vi "Update INI key to users last set value for Boolean.vi"(8 "error in (no error)":errorcluster, 9 "TF for INI (in)":bool, 10 "INI Key":string, 11 "INI Section":string) -> (0 "error out":errorcluster, 1 "TF for INI (out)":bool)   [LabVIEW 2010]
uses:
  <vilib>/Utility/sysdir.llb/System Directory Type.ctl
  <vilib>/Utility/config.llb/Write Key (Boolean).vi
  <vilib>/Utility/config.llb/NI_LVConfig.lvlib
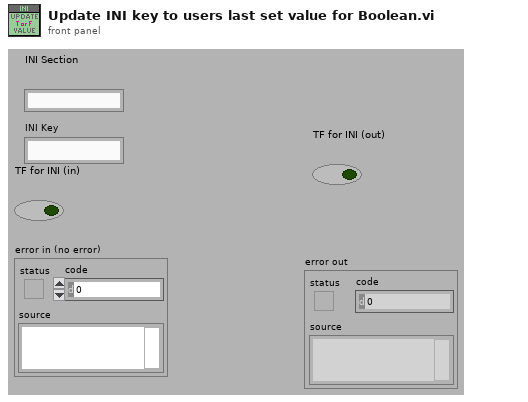
[diagram p1: front panel]
types:
  T1 = typedef "System Directory Type.ctl" = i32
  T2 = typedef "NI_LVConfig.lvlib/Config Data RefNum.ctl" = refnum<k1>
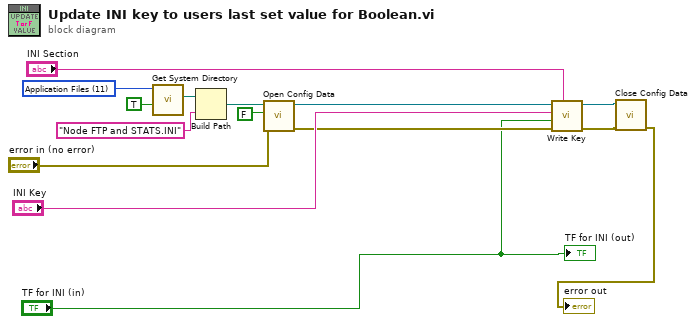
[diagram p0: block diagram]
diagram:
  w12 = T1 11 items=["User Home"=0, "User Desktop"=1, "User Documents"=2, "User Application Data"=3, "User Preferences"=4, "User Temporary"=5, "Public Documents"=6, "Public Application Data"=7, "Public Preferences"=8, "Public Cache"=13, "System Core Libraries"=9, "System Installed Libraries"=10, "Application Files"=11, "Boot Volume Root"=12] ("system directory type")
  n1 = call <vilib>:"Get System Directory.vi"("create directory if not found? (F)"=TRUE, "system directory type"=w12) -> ("system directory"=w11:path)  [unwired: 9 in]
  n2 = Build Path(base path=w11, name or relative path="Node FTP and STATS.INI") -> (appended path=w9:path)
  n3 = call <vilib>:"Open Config Data.vi"("error in (no error)"="error in (no error)", "create file if necessary (T)"=FALSE, "configuration file path"=w9) -> ("error out"=w5:errorcluster, "refnum"=w15:T2)  [unwired: 6 in, 1 out]
  n4 = call-poly <vilib>:"Write Key.vi"("section"="INI Section", "error in (no error)"=w5, "value"="TF for INI (in)", "key"="INI Key", "refnum"=w15) -> ("error out"=w4:errorcluster, "refnum out"=w8:T2)  [unwired: 4 in, 1 out]
  n5 = call <vilib>:"Close Config Data.vi"("error in (no error)"=w4, "refnum"=w8) -> ("error out"=→"error out":errorcluster)  [unwired: 8 in, 1 out]
  "TF for INI (out)" <- "TF for INI (in)"
